vi "Evaluate Part 1.vi"() -> ()   [LabVIEW 2021]
uses:
  Proto/Proto.lvclass
panel:
  out "size(s)":i32
  in  "Input":string
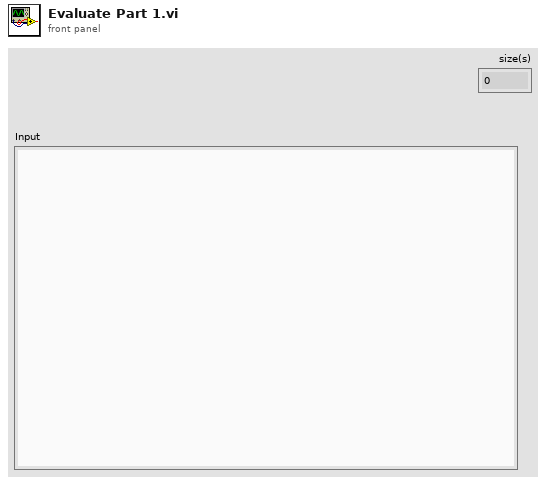
[diagram p1: front panel]
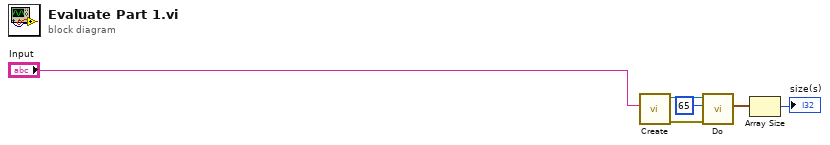
[diagram p0: block diagram]
diagram:
  n1 = call "Create.vi"("Input"="Input") -> ("error out"=w5:errorcluster, "Proto"=w6:refnum<class "Proto.lvclass">)  [unwired: 9 in]
  n2 = call "Do.vi"("error in (no error)"=w5, "Steps"=65, "Proto In"=w6) -> ("Possible Coords"=w2:cluster{"Row":i32, "Col":i32}[])  [unwired: 6 in, 2 out]
  n3 = Array Size(array=w2) -> (size(s)=→"size(s)":i32)
